vi "Get AccessToken.vi"(8 "error in (no error)":errorcluster, 11 "配置":T1={"url"="http://data.watersystem.com.cn:36091", "loginTokenRequest"={"clientId"="wqms_equip", "clientSecret"="2gJxw%vZkRGX8K7Se$^q", "grantType"="password", "password"="59315200", "scope"="read", "userName"="STDTEST001", "userType"="equip"}, "自动获取MN"=TRUE}) -> (0 "error out":errorcluster, 3 "response":T2)   [LabVIEW 2016, in "工况数据上传.lvlib"]
uses:
  <vilib>/httpClient/POSTBuffer.vi
  <vilib>/httpClient/LabVIEWHTTPClient.lvlib
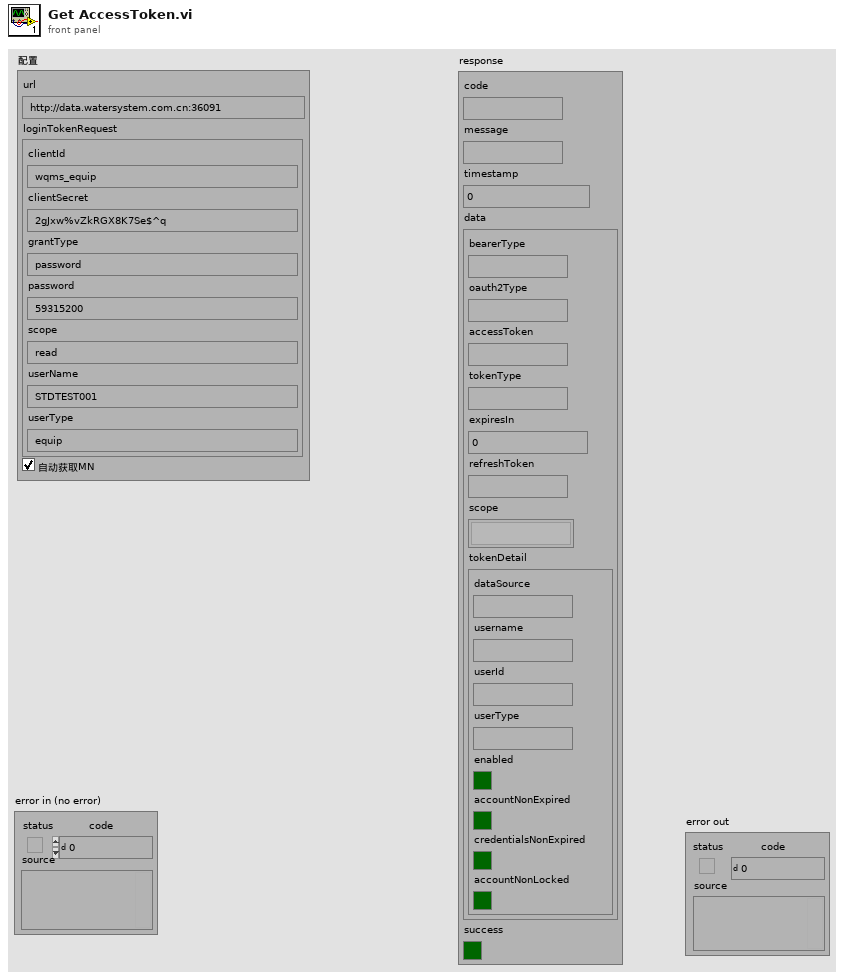
[diagram p1: front panel]
types:
  T1 = cluster{"url":string, "loginTokenRequest":cluster{"clientId":string, "clientSecret":string, "grantType":string, "password":string, "scope":string, "userName":string, "userType":string}, "自动获取MN":bool}
  T2 = cluster{"code":string, "message":string, "timestamp":u64, "data":cluster{"bearerType":string, "oauth2Type":string, "accessToken":string, "tokenType":string, "expiresIn":u64, "refreshToken":string, "scope":string[], "tokenDetail":cluster{"dataSource":string, "username":string, "userId":string, "userType":string, "enabled":bool, "accountNonExpired":bool, "credentialsNonExpired":bool, "accountNonLocked":bool}}, "success":bool}
  T3 = cluster{"code":string, "message":string, "timestamp":u64, "success":bool}
  T4 = cluster{"clientId":string, "clientSecret":string, "grantType":string, "password":string, "scope":string, "userName":string, "userType":string}
  T5 = typedef "LabVIEWHTTPClient.lvlib/ClientHandle.ctl" = refnum<k1>
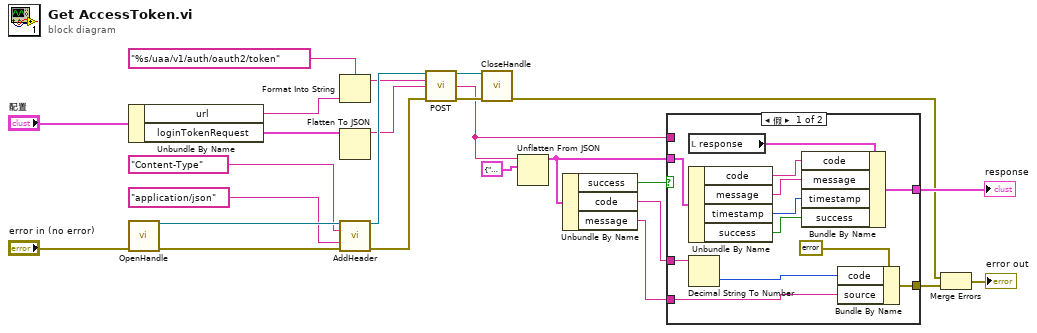
[diagram p0: block diagram]
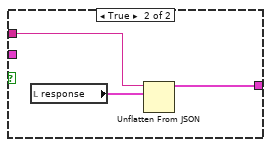
[diagram p2: hidden frame]
diagram:
  n1 = Unbundle By Name("配置") -> ("url"=w11:string, "loginTokenRequest"=w14:T4)
  n2 = call <vilib>:"OpenHandle.vi"("error in (no error)"="error in (no error)") -> ("client handle out"=w25:T5, "error out"=w23:errorcluster)  [unwired: 13 in]
  n3 = Format Into String(format string="%s/uaa/v1/auth/oauth2/token" ("url"), w11) -> (resulting string=w13:string)  [unwired: 2 in, 1 out]
  n4 = Flatten To JSON(anything=w14) -> (JSON string=w17:string)  [unwired: 2 in, 1 out]
  n5 = call <vilib>:"AddHeader.vi"("client handle"=w25, "header"="Content-Type", "value"="application/json", "error in (no error)"=w23) -> ("client handle out"=w21:T5, "error out"=w20:errorcluster)  [unwired: 10 in]
  n6 = call-poly <vilib>:"POST.vi"("client handle"=w21, "url"=w13, "buffer"=w17, "error in (no error)"=w20) -> ("client handle out"=w19:T5, "body"=w7:string, "error out"=w18:errorcluster)  [unwired: 8 in, 1 out]
  n7 = call <vilib>:"CloseHandle.vi"("client handle"=w19, "error in (no error)"=w18) -> ("error out"=w3:errorcluster)  [unwired: 13 in]
  n8 = Unflatten From JSON(JSON string=w7, type and defaults=T3 {"code"="", "message"="", "timestamp"=0, "success"=FALSE} ("response 2")) -> (value=w6:T3)  [unwired: 5 in, 1 out]
  n9 = Unbundle By Name(w6) -> ("success"=w9:bool, "code"=w1:string, "message"=w5:string)
  n10 = case shown="假" w9 {
    tunnel: [w36 w39] -> w8
    tunnel: w7 -> [_ w38]
    tunnel: w6 -> [w35 _]
    tunnel: w5 -> [w29 _]
    tunnel: [w28 _] -> w2
    tunnel: w1 -> [w27 _]
    frame False {
      n11 = local read "response"() -> (w37:T2)
      n12 = Unbundle By Name(w35) -> ("code"=w34:string, "message"=w33:string, "timestamp"=w32:u64, "success"=w31:bool)
      n13 = Decimal String To Number(string=w27) -> (number=w26:i32)  [unwired: 2 in, 1 out]
      n14 = Bundle By Name(cluster=w37, "code"=w34, "message"=w33, "timestamp"=w32, "success"=w31) -> (w36:T2)
      n15 = Bundle By Name(cluster=errorcluster {"status"=TRUE, "code"=0, "source"=""} ("错误常量"), "code"=w26, "source"=w29) -> (w28:errorcluster)
    }
    frame True {
      n16 = local read "response"() -> (w40:T2)
      n17 = Unflatten From JSON(JSON string=w38, type and defaults=w40) -> (value=w39:T2)  [unwired: 5 in, 1 out]
    }
  }
  "response" <- w8
  n18 = Merge Errors(w3, w2) -> (→"error out":errorcluster)
